vi "Register Cluster.vi"(7 "Package Name":string, 8 "error in":errorcluster, 10 "Cluster":variant, 11 "gRPCid in":T1) -> (0 "error out":errorcluster, 3 "gRPCid out":T1)   [LabVIEW 2019, in "grpc-lvsupport.lvlib"]
uses:
  grpc-lvsupport.lvlib
  grpcId.ctl
  <vilib>/Utility/error.llb/Error Cluster From Error Code.vi
  <resource>/libgrpc_labview.dll
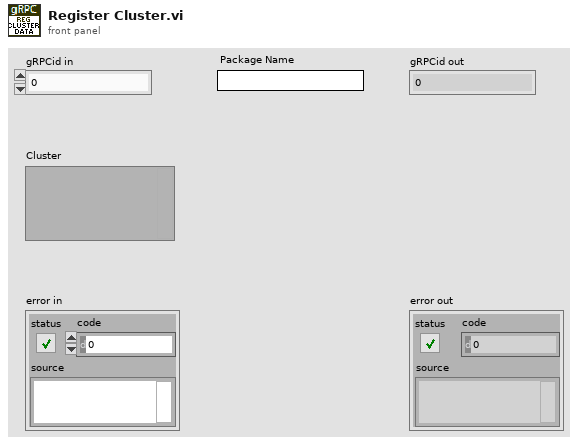
[diagram p1: front panel]
types:
  T1 = typedef "grpc-lvsupport.lvlib/grpcId.ctl" = u64
  T2 = typedef "grpc-lvsupport.lvlib/Message Metadata.ctl" = cluster{"Version":i32, "Name":string, "Type Url":string, "Elements":T3[], "Has Oneof":bool}
  T3 = typedef "grpc-lvsupport.lvlib/Message Element Metadata.ctl" = cluster{"Field Name":string, "Embedded Message Name":string, "Protobuf Index":i32, "MessageElementType":T4, "Repeated":bool, "Is in Oneof":bool, "Oneof Container Name":string}
  T4 = typedef "grpc-lvsupport.lvlib/Message Element Type.ctl" = enum32{"Int32Value", "FloatValue", "DoubleValue", "BoolValue", "StringValue", "MessageValue", "Int64Value", "UInt32Value", "UInt64Value", "EnumValue", "Bytes", "Fixed64", "Fixed32", "SFixed64", "SFixed32", "SInt64", "SInt32"}
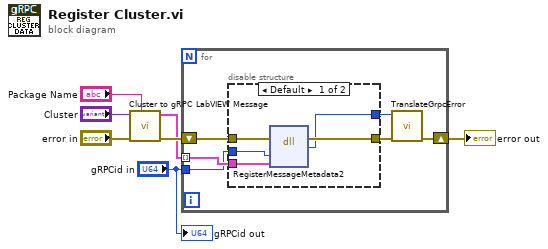
[diagram p0: block diagram]
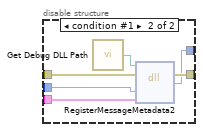
[diagram p2: hidden frame]
diagram:
  n1 = call "Cluster to gRPC LabVIEW Message.vi"("Package Name"="Package Name", "error in"="error in", "Cluster"="Cluster") -> ("error out"=w7:errorcluster, "gRPC Message Metadata []"=w6:T2[])  [unwired: 6 in, 1 out]
  n2 = for {
    tunnel: w6 -> [w11] mode=indexing
    shift-right: [w9] -> w2
    shift-left: w7 -> [w13]
    tunnel: "gRPCid in" -> [w10]
    n3 = disable-structure shown="Default" {
      disable-tunnel: w13 -> [w18 w24]
      disable-tunnel: [w17 w23] -> w12
      disable-tunnel: w11 -> [w16 w22]
      disable-tunnel: w10 -> [w15 w21]
      disable-tunnel: [w14 w20] -> w8
      frame condition #0 (active) {
        n4 = dll-call lib="C:/Program Files (x86)/National Instruments/LabVIEW 2024/resource/libgrpc_labview.*" fn="RegisterMessageMetadata2"(error in=w18, "serverId"=w15, "metadata"=w16) -> (error out=w17:errorcluster, "return type"=w14:i32)  [unwired: 4 in, 1 out]
      }
      frame condition #1 {
        n5 = call "Get Debug DLL Path.vi"() -> ("DLL Path"=w19:path)
        n6 = dll-call lib="?" fn="RegisterMessageMetadata2"(path in=w19, error in=w24, "serverId"=w21, "metadata"=w22) -> (error out=w23:errorcluster, "return type"=w20:i32)  [unwired: 3 in, 1 out]
      }
    }
    n7 = call "TranslateGrpcError.vi"("error in"=w12, "Error Code"=w8) -> ("error out"=w9:errorcluster)  [unwired: 9 in]
  }
  "error out" <- w2
  "gRPCid out" <- "gRPCid in"
